vi "Set Score.vi"(8 "error in (no error)":errorcluster, 10 "Score":T1, 11 "Submission in":refnum<class "Submission.lvclass">) -> (0 "error out":errorcluster, 3 "Submission out":refnum<class "Submission.lvclass">)   [LabVIEW 2020, in "Summer of LabVIEW.lvlib" / "Submission.lvclass"]
uses:
  Submission.lvclass
  Submission.lvclass/Submission.ctl
  SoL Scoring/Score Entry.ctl
  SoL Scoring/SoL Scoring.lvlib
  SoL Scoring/Score.ctl
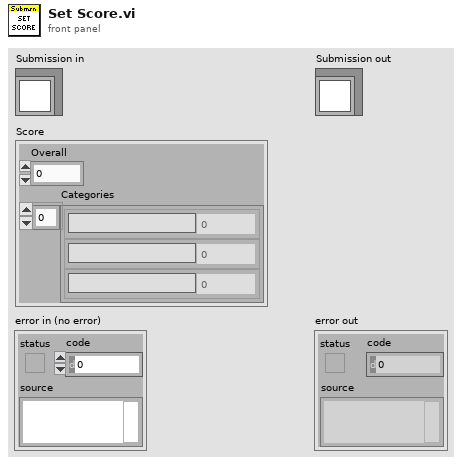
[diagram p1: front panel]
types:
  T1 = typedef "SoL Scoring.lvlib/Score.ctl" = cluster{"Overall":dbl, "Categories":T2[]}
  T2 = typedef "SoL Scoring.lvlib/Score Entry.ctl" = cluster{"Category":string, "Value":dbl}
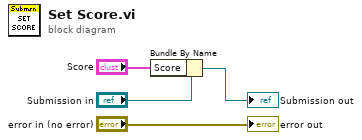
[diagram p0: block diagram]
diagram:
  n1 = Bundle By Name(cluster="Submission in", "Score"="Score") -> (→"Submission out":refnum<class "Submission.lvclass">)
  "error out" <- "error in (no error)"
